vi "EstimateTargetPostion.vi"(2 "Robot Y (in)":dbl, 3 "Robot X (in)":dbl) -> (0 "Estimated Heading to Target (deg)":dbl, 1 "Estimated Distance to Target (in)":dbl)   [LabVIEW 2019]
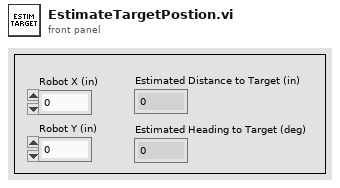
[diagram p1: front panel]
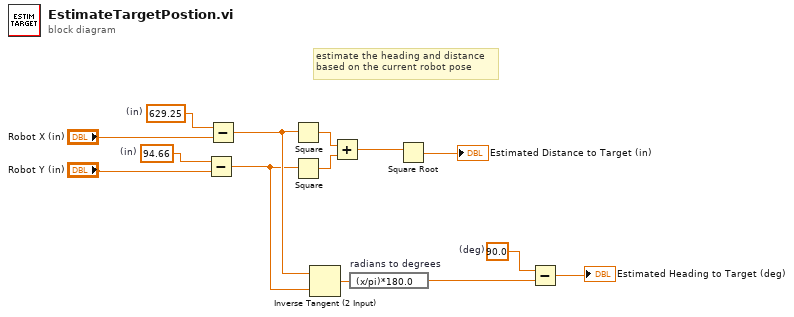
[diagram p0: block diagram]
diagram:
  w4 = 90.0  # (deg)
  w8 = 94.66  # (in)
  w10 = 629.25  # (in)
  # "estimate the heading and distance\nbased on the current robot pose"
  n1 = Subtract(x=w8, y="Robot Y (in)") -> (x-y=w5:dbl)
  n2 = Subtract(x=w10, y="Robot X (in)") -> (x-y=w6:dbl)
  n3 = Square(x=w6) -> (x^2=w14:dbl)
  n4 = Square(x=w5) -> (x^2=w13:dbl)
  n5 = Inverse Tangent (2 Input)(1:w5, 2:w6) -> (0:w2:dbl)
  n6 = Add(x=w14, y=w13) -> (x+y=w12:dbl)
  n7 = expression code="(x/pi)*180.0" "radians to degrees"(w2) -> (w1:dbl)
  n8 = Square Root(x=w12) -> (sqrt(x)=→"Estimated Distance to Target (in)":dbl)
  n9 = Subtract(x=w4, y=w1) -> (x-y=→"Estimated Heading to Target (deg)":dbl)
